vi "Results_plotter_Global.vi"() -> ()   [LabVIEW 2022 SP3]
uses:
  Data plotting/subVIs/Dispose_Channel.ctl
  RFP_Plot_Metadata.ctl
  Error_bars_index.ctl
panel:
  in  "Tab Control":T1(tab)
  in  "Plotted Raw data Filenames":string[](array[string])
  in  "Load number":i32
  in  "Plot EnFlo Tunnel Display":bool
  in  "Multi Ordinate?":bool
  out "Clear accept array":bool
  in  "Transpose":bool
  out "First Loop":bool
  out "Dispose of Chs?":bool
  in  "InterpolationStyle":T2(ring)=enum."Line"
  in  "TinyPoints?":bool
  in  "Max no of filter options":i32=2000
  in  "loadStartTime":timestamp format="%<%x %.3X>T"
  in  "Raw Data Filename index":i32
  in  "Row Reference":i32[][](array[numeric])
  in  "Plotted Row Numbers":i32[](array[numeric])
  in  "Scale":u16 min=1 max=10000 step=50
  in  "OutputType":enum16{"PDF", "PNG-ReportStyle"}(ring)
  in  "Units":enum16{"Metric", "English"}(ring)
  out "Data Dir":string[](array[string])
  in  "Results files Loaded":path[](array[path])
  in  "Setup Filename":string
  in  "Template":path
  in  "Current Data Filenames":string
  in  "Min plotted value":dbl
  in  "Max plotted value":dbl
  in  "All Template Ch Names":string[](array[string])
  out "Channel names":string[](array[string])
  out "Full Ch Names":string[](array[string])
  in  "3D Ch Names":string[](array[string])
  in  "3D Ch Selectors":i32[](array[numeric])
  out "Column Header String":string
  out "Filter 1 Strings":string[](array[string])
  out "Filter 2 Strings":string[](array[string])
  out "Filters 3 onwards":string[](array[string])
  out "Skip Dialog on these Channels":string[](array[string])
  out "Description":string[](array[string])
  in  "Dispose":T3[](array[typedef])
  out "Precision":string[](array[string])
  out "Summarise":string[](array[string])
  out "Tolerances":dbl[](array[numeric])
  out "Maths":string[](array[string])
  in  "Plot Metadata":T4[](array[typedef])
  out "Legend of ch names":string[](array[string])
  out "Legend":string[](array[string])
  out "Ordinate Strings":string[](array[string])
  in  "Series Index":i32[](array[numeric])
  in  "Value plotted Name":string
  in  "Y Axis Name":string
  in  "X Axis Name":string
  out "Plot Summary":string[][](array[string])
  out "legendExpansion":dbl
  out "Point info":T6(array[cluster])
  out "X Scale":cluster{"Xo":dbl, "delta X":dbl} {"delta X" format="%.2f"; "Xo" format="%.2f"}
  out "Y Scale":cluster{"Xo":dbl, "delta X":dbl} {"delta X" format="%.2f"; "Xo" format="%.2f"}
  in  "X plot min":dbl
  in  "X plot max":dbl
  in  "Y plot min":dbl
  in  "Y plot max":dbl
  out "Z Max":dbl format="%.2f"
  out "Z Min":dbl format="%.2f"
  out "Max Values":string[](array[string])
  out "Min Values":string[](array[string])
  out "Absisca":i32
  out "Ordinate":i32[](array[numeric])
  out "Y Max":dbl format="%.2f"
  out "X Max":dbl format="%.2f"
  out "Raw Interpolation":dbl[][](array[numeric]) format="%.2f"
  in  "Surface Integral":dbl format="%.2f"
  in  "Surface Area":dbl format="%.2f"
  out "Intensity Plot data in rows":dbl[][](array[numeric]) format="%.2f"
  in  "Error_bars_index":T5
  in  "X Values":dbl[](array[numeric]) format="%.2f"
  in  "Y Values":dbl[](array[numeric]) format="%.2f"
  in  "New Chs In":string[](array[string])
  in  "New Values In":string[][](array[string])
  in  "New Values Row index":i32[](array[numeric])
  in  "3DgiveUp":bool
  out "3DvectorFieldSDRadius":dbl
  out "3DvectorFieldMeanRadius":dbl
  out "3DvectorMedian":cluster{"X":sgl, "Y":sgl, "Z":sgl}
  # "File Num       RowInFile     RowInPlotter"
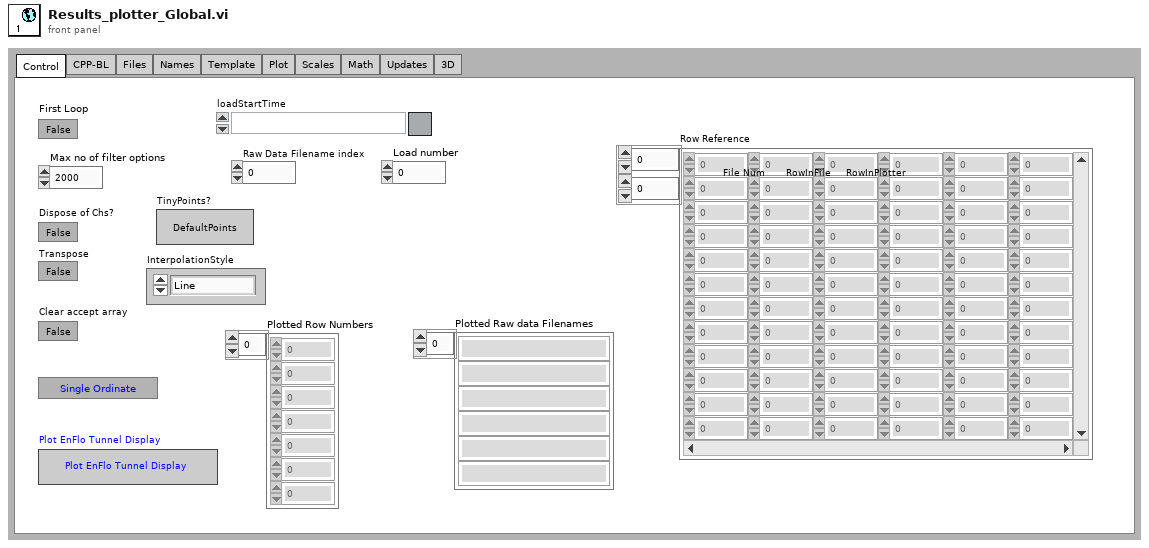
[diagram p1: front panel]
types:
  T1 = enum32{"Control", "CPP-BL", "Files", "Names", "Template", "Plot", "Scales", "Math", "Updates", "3D"}
  T2 = enum16{"Points", "StepLeft", "Line", "StepRight", "StepCentre", "StepEdge"}
  T3 = typedef "Dispose_Channel.ctl" = enum16{"Always", "If Blank", "Never"}
  T4 = typedef "RFP_Plot_Metadata.ctl" = cluster{"Row Number":i32[], "Error Bars":T5, "X Label":string, "Y Label":string, "Blanks NaNs":i32[]}
  T5 = typedef "Error_bars_index.ctl" = cluster{"Upper":i32, "Lower":i32, "St Error":i32}
  T6 = cluster{"Plot Color":u32, "Plot Interpolation":u8, "Point Style":u8, "Line Style":u8, "Fill/Pt. Color":u32, "Line Width":u8, "Bar Plot Style":u8, "Fill To":i16}[]
diagram:
